vi "Кнопка побег и размер.vi"() -> ()   [LabVIEW 2021]
uses:
  <vilib>/Utility/miscctls.llb/LVPositionTypeDef.ctl
panel:
  in  "stop 2":bool
  in  "Буги/Следуй":bool
  out "LED":bool
  out "result":T1
  out "Position 2":T1
  out "Position":T1
  out "x*y":T1
  in  "Определить размер \nкнопки по \nDefault":bool
  in  "Изменить\n размер":bool
  in  "stop":bool
  in  "Вкл":bool
  # "Нажать еще раз,\n чтобы сработало"
types:
  T1 = typedef "LVPositionTypeDef.ctl" = cluster{"Left":i32, "Top":i32}
  T2 = typedef "LVPoint32TypeDef.ctl" = cluster{"Horizontal":i32, "Vertical":i32}
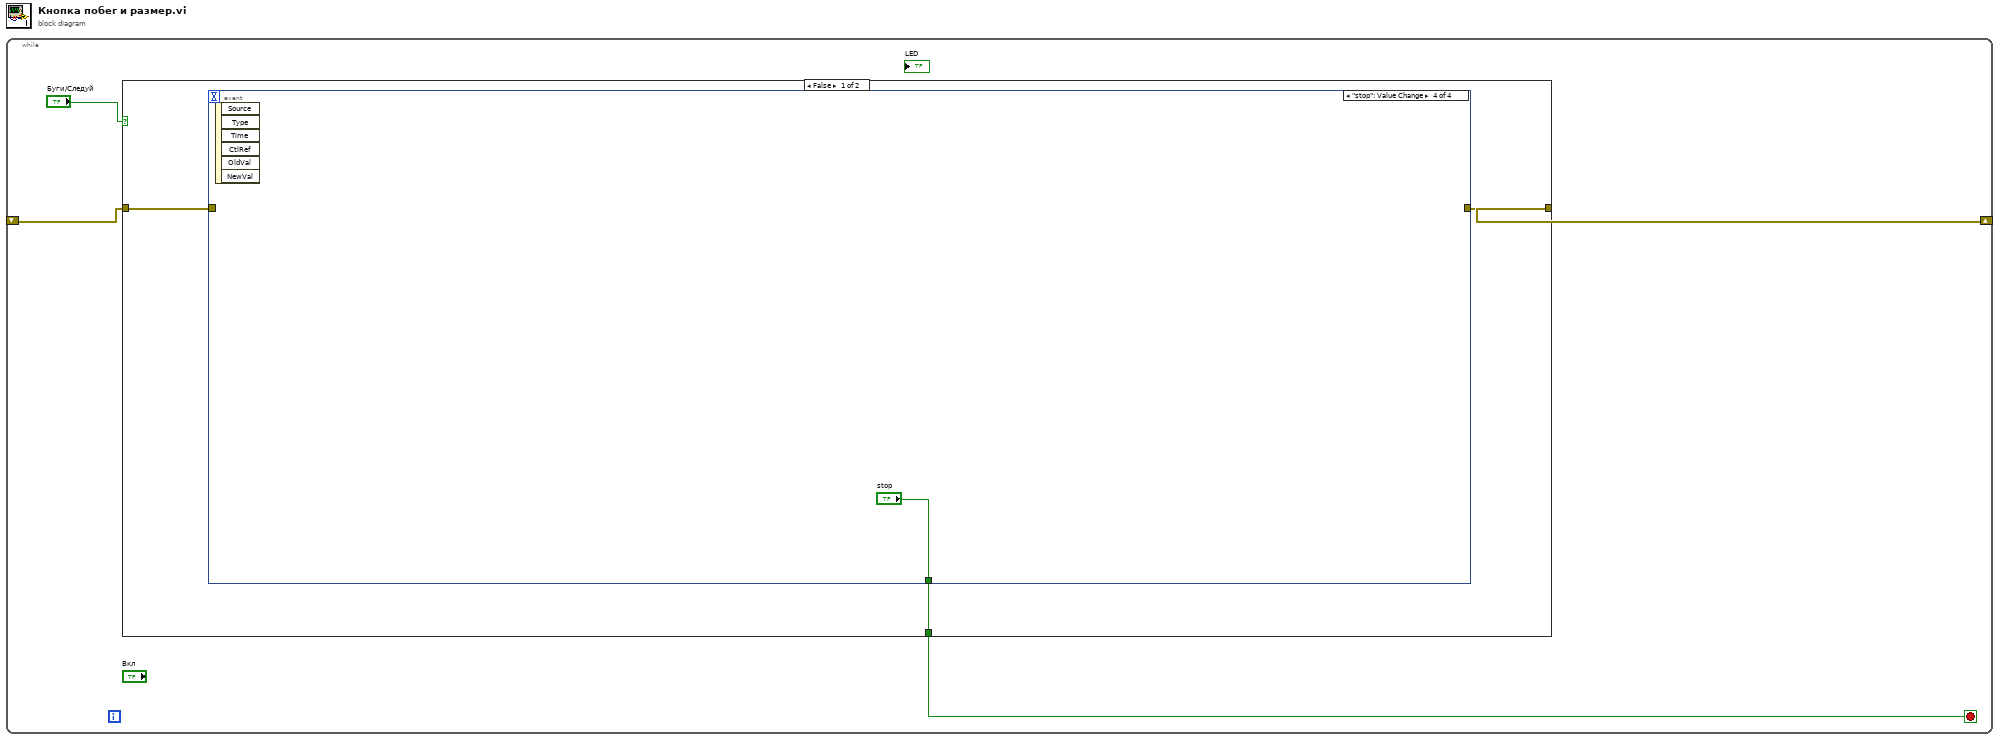
[diagram p0: block diagram]
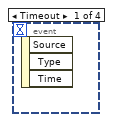
[diagram p2: hidden frame]
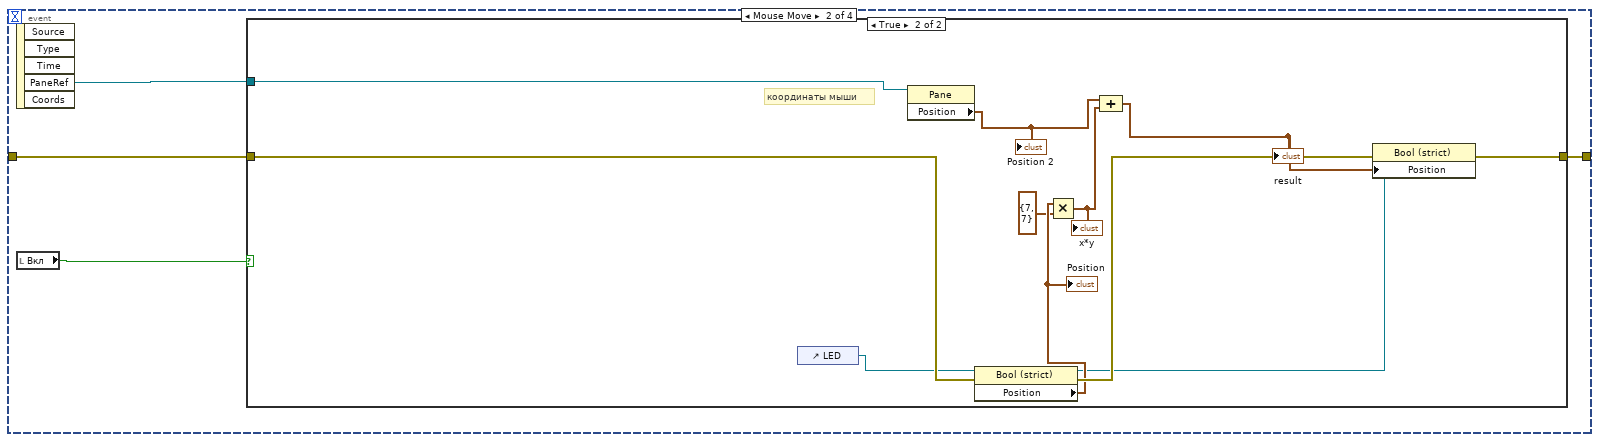
[diagram p3: hidden frame]
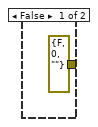
[diagram p4: hidden frame]
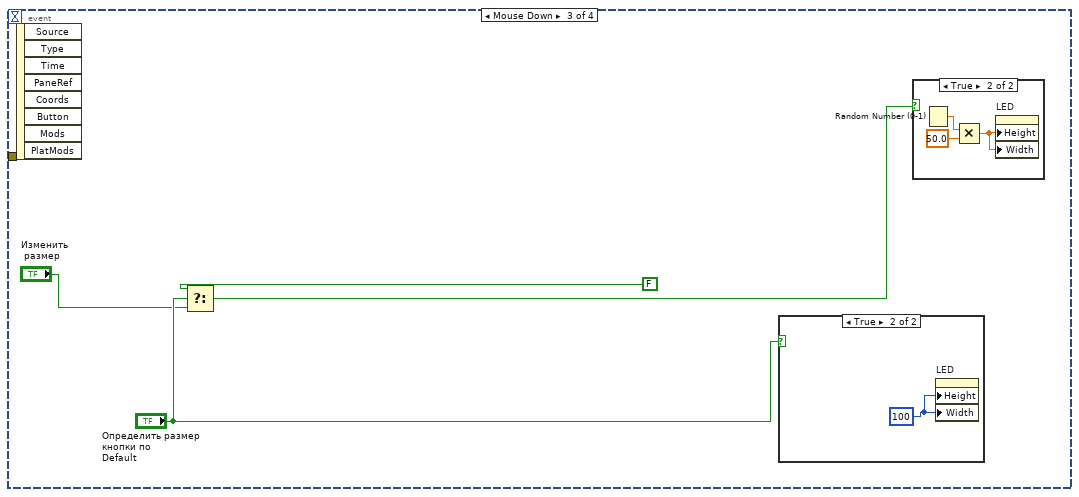
[diagram p5: hidden frame]
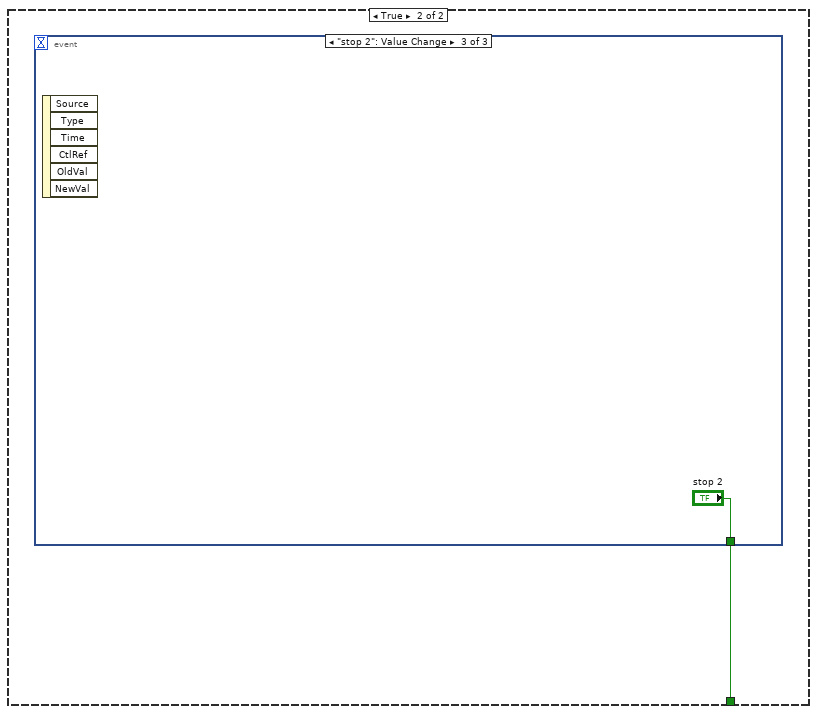
[diagram p8: hidden frame]
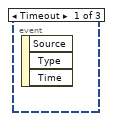
[diagram p9: hidden frame]
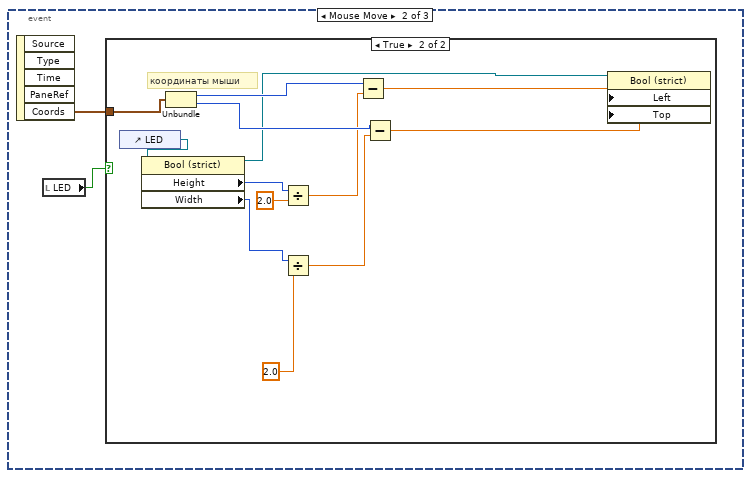
[diagram p10: hidden frame]
diagram:
  n1 = while {
    shift-right: [w3] -> _
    shift-left: _ -> [w4]
    stop <- w1 stop-if-true
    n2 = case shown="False" "Буги/Следуй" {
      tunnel: w4 -> [w7 _]
      tunnel: [w6 _] -> w3
      tunnel: [w5 w33] -> w1
      frame False {
        n3 = event shown="[3] \"stop\": Value Change" {
          selector: _ -> [_ _ _ _]
          dyn-events: _ -> [_ _ _ _]
          timeout: _ -> [_ _ _ _]
          tunnel: [_ w10 _ _] -> w6
          tunnel: w7 -> [_ w9 _ _]
          tunnel: [_ _ _ "stop"] -> w5
          event Timeout {
            n4 = event-data() -> ()  [unwired: 1 in, 3 out]
          }
          event Mouse Move {
            n5 = event-data() -> ("PaneRef"=w8:refnum<vi>)  [unwired: 1 in, 4 out]
            n6 = local read "Вкл"() -> (w11:bool)
            n7 = case shown="True" w11 {
              tunnel: [errorcluster {"status"=FALSE, "code"=0, "source"=""} ("error out") w22] -> w10
              tunnel: w9 -> [_ w21]
              tunnel: w8 -> [_ w16]
              frame False {
              }
              frame True {
                # "координаты мыши"
                n8 = control-ref of="LED"() -> (w13:refnum<vi>)
                n9 = property class="Pane"(reference=w16) -> ("Position"=w15:T1)  [unwired: 1 in, 2 out]
                "Position 2" <- w15
                n10 = property class="Bool (strict)"(reference=w13, error in=w21) -> (reference out=w14:refnum<vi>, error out=w23:errorcluster, "Position"=w19:T1)
                "Position" <- w19
                n11 = Multiply(x=w19, y=T1 {"Left"=7, "Top"=7}) -> (x*y=w17:T1)
                "x*y" <- w17
                n12 = Compound Arithmetic op=ADD(w15, w17) -> (w20:T1)
                "result" <- w20
                n13 = property class="Bool (strict)"(reference=w14, error in=w23, "Position"=w20) -> (error out=w22:errorcluster)  [unwired: 1 out]
              }
            }
          }
          event Mouse Down {
            n14 = event-data() -> ()  [unwired: 1 in, 8 out]
            n15 = Select(t=FALSE ("Изменить\n размер"), s="Определить размер \nкнопки по \nDefault", f="Изменить\n размер") -> (s? t:f=w24:bool)
            n16 = case shown="True" "Определить размер \nкнопки по \nDefault" {
              frame False {
              }
              frame True {
                w28 = u32 100 ("Button Size:Height")
                n17 = property on="LED" class="Bool (strict)"("Height"=w28, "Width"=w28) -> ()  [unwired: 2 in, 2 out]
              }
            }
            n18 = case shown="True" w24 {
              frame False {
              }
              frame True {
                n19 = Random Number (0-1)() -> (number: 0 to 1=w31:dbl)
                n20 = Multiply(x=w31, y=50.0) -> (x*y=w29:dbl)
                n21 = property on="LED" class="Bool (strict)"("Height"=w29, "Width"=w29) -> ()  [unwired: 2 in, 2 out]
              }
            }
          }
          event "stop": Value Change {
            n22 = event-data() -> ()  [unwired: 1 in, 6 out]
          }
        }
      }
      frame True {
        n23 = event shown="[2] \"stop 2\": Value Change" {
          selector: _ -> [_ _ _]
          dyn-events: _ -> [_ _ _]
          timeout: _ -> [_ _ _]
          tunnel: [_ _ "stop 2"] -> w33
          event Timeout {
            n24 = event-data() -> ()  [unwired: 1 in, 3 out]
          }
          event Mouse Move {
            n25 = event-data() -> ("Coords"=w35:T2)  [unwired: 1 in, 4 out]
            n26 = local read "LED"() -> (w34:bool)
            n27 = case shown="True" w34 {
              tunnel: w35 -> [_ w48]
              frame False {
              }
              frame True {
                # "координаты мыши"
                n28 = control-ref of="LED"() -> (w37:refnum<vi>)
                n29 = property on="Property Node" class="Bool (strict)"(reference=w37) -> (reference out=w36:refnum<vi>, "Height"=w44:u32, "Width"=w45:u32)  [unwired: 1 in, 1 out]
                n30 = Unbundle(w48) -> ("Horizontal"=w43:i32, "Vertical"=w42:i32)
                n31 = Divide(x=w44, y=2.0) -> (x/y=w40:dbl)
                n32 = Divide(x=w45, y=2.0) -> (x/y=w41:dbl)
                n33 = Subtract(x=w43, y=w40) -> (x-y=w39:dbl)
                n34 = Subtract(x=w42, y=w41) -> (x-y=w38:dbl)
                n35 = property on="Property Node" class="Bool (strict)"(reference=w36, "Left"=w39, "Top"=w38) -> ()  [unwired: 1 in, 2 out]
              }
            }
          }
          event "stop 2": Value Change {
            n36 = event-data() -> ()  [unwired: 1 in, 6 out]
          }
        }
      }
    }
  }
